vi "Sans titre 5.vi"() -> ()   [LabVIEW 2020]
uses:
  <vilib>/addons/database/Connection.llb/DB Tools Open Connec (String).vi
  <vilib>/addons/database/Connection.llb/Conn Execute.vi
  <vilib>/addons/database/Recordset.llb/Rec Fetch Recordset Data (R).vi
  <vilib>/addons/database/Recordset.llb/Rec Destroy - Connection.vi
  <vilib>/addons/database/NI_Database_API.lvlib
panel:
  out "Cluster":T1
  out "données":string[](array[string])
  out "recordset data":variant[][](array[variant])
  in  "errin":errorcluster
  in  "type":string
  out "error out":errorcluster
  in  "Limites de test":T1
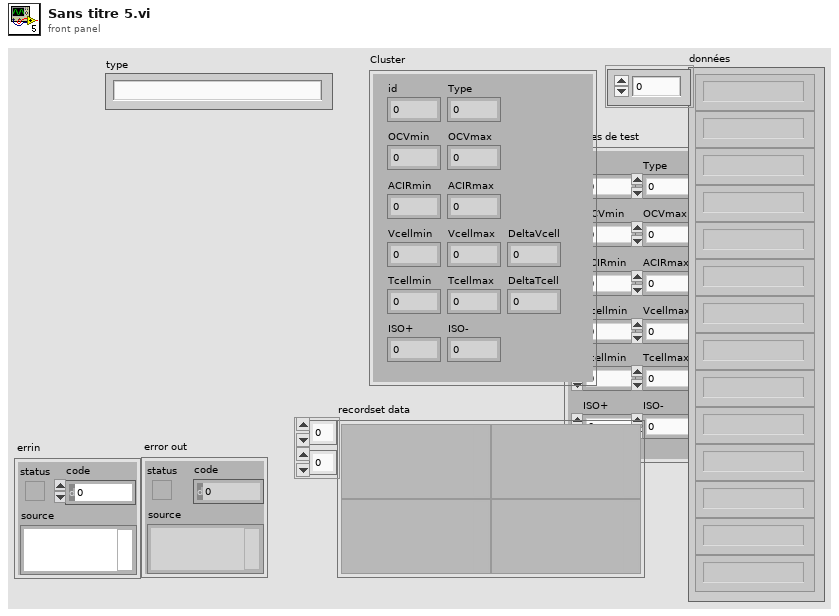
[diagram p1: front panel]
types:
  T1 = cluster{"id":dbl, "Type":dbl, "OCVmin":dbl, "OCVmax":dbl, "ACIRmin":dbl, "ACIRmax":dbl, "Vcellmin":dbl, "Vcellmax":dbl, "DeltaVcell":dbl, "Tcellmin":dbl, "Tcellmax":dbl, "DeltaTcell":dbl, "ISO+":dbl, "ISO-":dbl}
  T2 = typedef "NI_Database_API.lvlib/Conn ObjectReference.ctl" = refnum<k1>
  T3 = typedef "NI_Database_API.lvlib/Rec ObjectReference.ctl" = refnum<k1>
  T4 = cluster{"[0]":dbl, "[1]":dbl, "[2]":dbl, "[3]":dbl, "[4]":dbl, "[5]":dbl, "[6]":dbl, "[7]":dbl, "[8]":dbl, "[9]":dbl, "[10]":dbl, "[11]":dbl, "[12]":dbl, "[13]":dbl}
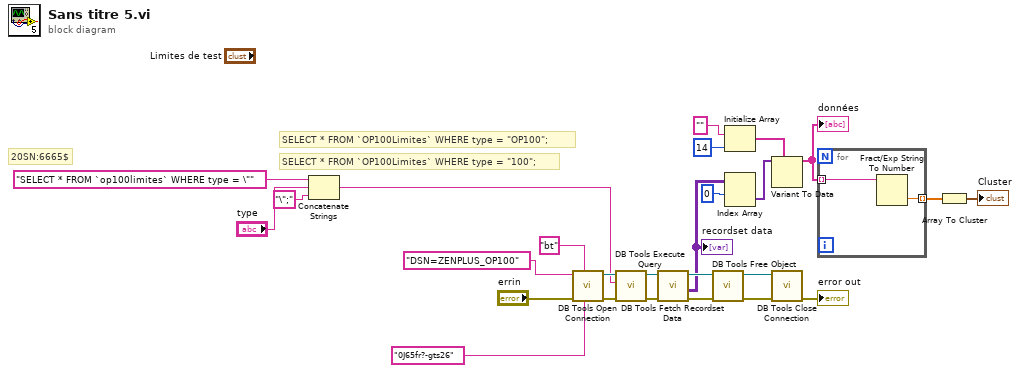
[diagram p0: block diagram]
diagram:
  # "SELECT * FROM `OP100Limites` WHERE type = \"OP100\";"
  # "SELECT * FROM `OP100Limites` WHERE type = \"100\";"
  # "20SN:6665$"
  n1 = Concatenate Strings("SELECT * FROM `op100limites` WHERE type = \"" ("SQL query"), "type", "\";" ("chaîne")) -> (w14:string)
  n2 = call-poly <vilib>:"DB Tools Open Connection.vi"("password"="0J65fr?-gts26", "userID"="bt", "error in (no error)"="errin", "connection information"="DSN=ZENPLUS_OP100") -> ("error out"=w26:errorcluster, "connection reference"=w24:T2)  [unwired: 4 in]
  n3 = call-poly <vilib>:"DB Tools Execute Query.vi"("error in (no error)"=w26, "SQL query"=w14, "connection reference"=w24) -> ("error out"=w19:errorcluster, "recordset reference"=w18:T3)  [unwired: 5 in]
  n4 = call-poly <vilib>:"DB Tools Fetch Recordset Data.vi"("error in (no error)"=w19, "recordset reference"=w18) -> ("error out"=w20:errorcluster, "recordset data"=w11:variant[][], "recordset reference out"=w17:T3)  [unwired: 3 in]
  "recordset data" <- w11
  n5 = call-poly <vilib>:"DB Tools Free Object.vi"("error in (no error)"=w20, "recordset reference"=w17) -> ("error out"=w25:errorcluster, "connection reference"=w23:T2)  [unwired: 8 in]
  n6 = Initialize Array("", 14 ("taille de la dimension")) -> (w7:string[])
  n7 = Index Array(array=w11, index (row)=0 ("indice (ligne)")) -> (element=w9:variant[])  [unwired: 1 in]
  n8 = Variant To Data ("Variant en donnée")(type=w7, Variant=w9) -> (data=w6:string[])  [unwired: 1 in, 1 out]
  "données" <- w6
  n9 = call <vilib>:"DB Tools Close Connection.vi"("error in (no error)"=w25, "connection reference"=w23) -> ("error out"=→"error out":errorcluster)  [unwired: 5 in]
  n10 = for {
    tunnel: w6 -> [w28] mode=indexing
    tunnel: [w27] -> w5 mode=indexing
    n11 = Fract/Exp String To Number(string=w28) -> (number=w27:dbl)  [unwired: 3 in, 1 out]
  }
  n12 = Array To Cluster ("Tableau en cluster")(array=w5) -> (cluster=→"Cluster":T4)
